vi "Lab Panel V5.25.vi"() -> ()   [LabVIEW 2017] (continued)
                            n3233 = Multiply(x=w5970, y=w5972) -> (x*y=w5971:dbl)
                          }
                        }
                        n3234 = local read "SIG LAB05-1"() -> (w5957:T2)
                        n3235 = Bundle By Name(cluster=w5957, "Tmp Live"=w5937, "Tmp Neut"=w5936) -> (w5956:T2)
                        n3236 = local read "SIG LAB05-2"() -> (w5955:T2)
                        n3237 = Bundle By Name(cluster=w5955, "Tmp Live"=w5933, "Tmp Neut"=w5932) -> (w5954:T2)
                        n3238 = local write "SIG LAB05-1"(w5956) -> ()
                        n3239 = local write "SIG LAB05-2"(w5954) -> ()
                      }
                    }
                  }
                }
              }
            }
          }
          frame #21 {
            # "write data to display panel"
            n3240 = global write "Global display 1.vi" "TEST 5-2"(w6009) -> ()
            n3241 = global write "Global display 1.vi" "TEST 4-2"(w6011) -> ()
            n3242 = global write "Global display 1.vi" "TEST 1-2"(w6017) -> ()
            n3243 = global write "Global display 1.vi" "TEST 3-1"(w6014) -> ()
            n3244 = global write "Global display 1.vi" "TEST 5-1"(w6010) -> ()
            n3245 = global write "Global display 1.vi" "TEST 1-1"(w6018) -> ()
            n3246 = global write "Global display 1.vi" "TEST 3-2"(w6013) -> ()
            n3247 = global write "Global display 1.vi" "TEST 4-1"(w6012) -> ()
            n3248 = global write "Global display 1.vi" "TEST 2-2"(w6015) -> ()
            n3249 = global write "Global display 1.vi" "TEST 2-1"(w6016) -> ()
            n3250 = global read "Global display 3.vi" "log 1-1"() -> (→"LOG LAB01-1":string)
            n3251 = global read "Global display 3.vi" "log 3-1"() -> (→"LOG LAB03-1":string)
            n3252 = global read "Global display 3.vi" "log 1-2"() -> (→"LOG LAB01-2":string)
            n3253 = property on="Tab Control 2" class="TabCtl (strict)"() -> ("Pages"=w6008:refnum<vi>[])  [unwired: 2 in, 2 out]
            n3254 = global read "Global display 3.vi" "log 2-1"() -> (→"LOG LAB02-1":string)
            n3255 = global read "Global display 3.vi" "log 2-2"() -> (→"LOG LAB02-2":string)
            n3256 = global read "Global display 3.vi" "log 4-2"() -> (→"LOG LAB04-2":string)
            n3257 = global read "Global display 3.vi" "log 5-2"() -> (→"LOG LAB05-2":string)
            n3258 = global read "Global display 3.vi" "log 5-1"() -> (→"LOG LAB05-1":string)
            n3259 = global read "Global display 3.vi" "log 4-1"() -> (→"LOG LAB04-1":string)
            n3260 = global read "Global display 3.vi" "log 3-2"() -> (→"LOG LAB03-2":string)
            n3261 = Index Array(array=w6008, index=8) -> (element=w6006:refnum<vi>)
            n3262 = property class="Page"(reference=w6006) -> ("PageVis"=w6005:bool)  [unwired: 1 in, 2 out]
            n3263 = global write "Global display 3.vi" "admin"(w6005) -> ()
            n3264 = local read "O/I  LAB05-2"() -> (w6059:bool)
            n3265 = local read "O/I  LAB05-1"() -> (w6060:bool)
            n3266 = local read "O/I  LAB03-2"() -> (w6063:bool)
            n3267 = local read "O/I  LAB04-2"() -> (w6061:bool)
            n3268 = local read "O/I  LAB04-1"() -> (w6062:bool)
            n3269 = local read "O/I  LAB03-1"() -> (w6064:bool)
            n3270 = local read "O/I  LAB01-2"() -> (w6067:bool)
            n3271 = local read "O/I  LAB01-1"() -> (w6068:bool)
            n3272 = local read "O/I  LAB02-1"() -> (w6066:bool)
            n3273 = local read "O/I  LAB02-2"() -> (w6065:bool)
            n3274 = global write "Global display 1.vi" "5-2 O/F"(w6059) -> ()
            n3275 = global write "Global display 1.vi" "5-1 O/F"(w6060) -> ()
            n3276 = global write "Global display 1.vi" "4-1 O/F"(w6062) -> ()
            n3277 = global write "Global display 1.vi" "4-2 O/F"(w6061) -> ()
            n3278 = global write "Global display 1.vi" "3-2 O/F"(w6063) -> ()
            n3279 = global write "Global display 1.vi" "3-1 O/F"(w6064) -> ()
            n3280 = global write "Global display 1.vi" "2-2 O/F"(w6065) -> ()
            n3281 = global write "Global display 1.vi" "2-1 O/F"(w6066) -> ()
            n3282 = global write "Global display 1.vi" "1-2 O/F"(w6067) -> ()
            n3283 = global write "Global display 1.vi" "1-1 O/F"(w6068) -> ()
            n3284 = local read "run lab05-2"() -> (w6049:bool)
            n3285 = local read "run lab04-1"() -> (w6052:bool)
            n3286 = local read "run lab04-2"() -> (w6051:bool)
            n3287 = local read "run lab05-1"() -> (w6050:bool)
            n3288 = local read "TEMP START LAB02-2"() -> (w5991:cluster{"TL":dbl, "TN":dbl})
            n3289 = local read "TEMP START LAB01-2"() -> (w5993:cluster{"TL":dbl, "TN":dbl})
            n3290 = local read "TEMP START LAB02-1"() -> (w5992:cluster{"TL":dbl, "TN":dbl})
            n3291 = local read "TEMP START LAB04-1"() -> (w5988:cluster{"TL":dbl, "TN":dbl})
            n3292 = local read "TEMP START LAB04-2"() -> (w5987:cluster{"TL":dbl, "TN":dbl})
            n3293 = local read "run lab03-2"() -> (w6053:bool)
            n3294 = local read "TEMP START LAB01-1"() -> (w5994:cluster{"TL":dbl, "TN":dbl})
            n3295 = local read "TEMP START LAB05-2"() -> (w5985:cluster{"TL":dbl, "TN":dbl})
            n3296 = local read "TEMP START LAB05-1"() -> (w5986:cluster{"TL":dbl, "TN":dbl})
            n3297 = local read "run lab02-1"() -> (w6056:bool)
            n3298 = local read "run lab03-1"() -> (w6054:bool)
            n3299 = local read "TEMP START LAB03-2"() -> (w5989:cluster{"TL":dbl, "TN":dbl})
            n3300 = local read "run lab01-2"() -> (w6057:bool)
            n3301 = local read "run lab02-2"() -> (w6055:bool)
            n3302 = local read "TEMP START LAB03-1"() -> (w5990:cluster{"TL":dbl, "TN":dbl})
            n3303 = local read "run lab01-1"() -> (w6058:bool)
            n3304 = global write "Global display 1.vi" "5-2 R/S"(w6049) -> ()
            n3305 = global write "Global display 1.vi" "5-1 R/S"(w6050) -> ()
            n3306 = global write "Global display 1.vi" "4-2 R/S"(w6051) -> ()
            n3307 = global write "Global display 1.vi" "4-1 R/S"(w6052) -> ()
            n3308 = global write "Global display 1.vi" "3-2 R/S"(w6053) -> ()
            n3309 = global write "Global display 1.vi" "1-2 R/S"(w6057) -> ()
            n3310 = global write "Global display 1.vi" "2-1 R/S"(w6056) -> ()
            n3311 = global write "Global display 1.vi" "3-1 R/S"(w6054) -> ()
            n3312 = global write "Global display 1.vi" "2-2 R/S"(w6055) -> ()
            n3313 = global write "Global display 1.vi" "1-1 R/S"(w6058) -> ()
            n3314 = global write "Global display 3.vi" "TEMP ST 05-2"(w5985) -> ()
            n3315 = global write "Global display 3.vi" "TEMP ST 05-1"(w5986) -> ()
            n3316 = global write "Global display 3.vi" "TEMP ST 03-2"(w5989) -> ()
            n3317 = global write "Global display 3.vi" "TEMP ST 04-2"(w5987) -> ()
            n3318 = global write "Global display 3.vi" "TEMP ST 01-1"(w5994) -> ()
            n3319 = global write "Global display 3.vi" "TEMP ST 01-2"(w5993) -> ()
            n3320 = global write "Global display 3.vi" "TEMP ST 04-1"(w5988) -> ()
            n3321 = global write "Global display 3.vi" "TEMP ST 02-1"(w5992) -> ()
            n3322 = global write "Global display 3.vi" "TEMP ST 02-2"(w5991) -> ()
            n3323 = global write "Global display 3.vi" "TEMP ST 03-1"(w5990) -> ()
            n3324 = local read "DISP LAB04-2"() -> (w6041:T4)
            n3325 = local read "DISP LAB05-1"() -> (w6040:T4)
            n3326 = local read "DISP LAB04-1"() -> (w6042:T4)
            n3327 = local read "DISP LAB05-2"() -> (w6039:T4)
            n3328 = local read "DISP LAB03-1"() -> (w6044:T4)
            n3329 = local read "DISP LAB03-2"() -> (w6043:T4)
            n3330 = local read "DISP LAB01-2"() -> (w6047:T4)
            n3331 = local read "DISP LAB02-1"() -> (w6046:T4)
            n3332 = local read "DISP LAB02-2"() -> (w6045:T4)
            n3333 = local read "DISP LAB01-1"() -> (w6048:T4)
            n3334 = local read "TEMP RISE LAB05-1"() -> (w5976:cluster{"TL":dbl, "TN":dbl})
            n3335 = local read "TEMP RISE LAB05-2"() -> (w5975:cluster{"TL":dbl, "TN":dbl})
            n3336 = local read "TEMP RISE LAB04-2"() -> (w5977:cluster{"TL":dbl, "TN":dbl})
            n3337 = local read "TEMP RISE LAB04-1"() -> (w5978:cluster{"TL":dbl, "TN":dbl})
            n3338 = local read "TEMP RISE LAB03-2"() -> (w5979:cluster{"TL":dbl, "TN":dbl})
            n3339 = local read "TEMP RISE LAB03-1"() -> (w5980:cluster{"TL":dbl, "TN":dbl})
            n3340 = local read "TEMP RISE LAB01-2"() -> (w5983:cluster{"TL":dbl, "TN":dbl})
            n3341 = local read "TEMP RISE LAB02-2"() -> (w5981:cluster{"TL":dbl, "TN":dbl})
            n3342 = local read "TEMP RISE LAB01-1"() -> (w5984:cluster{"TL":dbl, "TN":dbl})
            n3343 = local read "TEMP RISE LAB02-1"() -> (w5982:cluster{"TL":dbl, "TN":dbl})
            n3344 = global write "Global display 2.vi" "DISP LAB05-1"(w6040) -> ()
            n3345 = global write "Global display 2.vi" "DISP LAB05-2"(w6039) -> ()
            n3346 = global write "Global display 2.vi" "DISP LAB04-2"(w6041) -> ()
            n3347 = global write "Global display 2.vi" "DISP LAB02-1"(w6046) -> ()
            n3348 = global write "Global display 2.vi" "DISP LAB02-2"(w6045) -> ()
            n3349 = global write "Global display 2.vi" "DISP LAB04-1"(w6042) -> ()
            n3350 = global write "Global display 2.vi" "DISP LAB01-2"(w6047) -> ()
            n3351 = global write "Global display 2.vi" "DISP LAB01-1"(w6048) -> ()
            n3352 = global write "Global display 2.vi" "DISP LAB03-1"(w6044) -> ()
            n3353 = global write "Global display 2.vi" "DISP LAB03-2"(w6043) -> ()
            n3354 = global write "Global display 3.vi" "TEMP RS 05-2"(w5975) -> ()
            n3355 = global write "Global display 3.vi" "TEMP RS 05-1"(w5976) -> ()
            n3356 = global write "Global display 3.vi" "TEMP RS 03-2"(w5979) -> ()
            n3357 = global write "Global display 3.vi" "TEMP RS 02-1"(w5982) -> ()
            n3358 = global write "Global display 3.vi" "TEMP RS 02-2"(w5981) -> ()
            n3359 = global write "Global display 3.vi" "TEMP RS 04-2"(w5977) -> ()
            n3360 = global write "Global display 3.vi" "TEMP RS 01-2"(w5983) -> ()
            n3361 = global write "Global display 3.vi" "TEMP RS 03-1"(w5980) -> ()
            n3362 = global write "Global display 3.vi" "TEMP RS 04-1"(w5978) -> ()
            n3363 = global write "Global display 3.vi" "TEMP RS 01-1"(w5984) -> ()
            n3364 = local read "SET LAB05-2"() -> (w6029:T5)
            n3365 = local read "SET LAB05-1"() -> (w6030:T5)
            n3366 = local read "SET LAB04-1"() -> (w6032:T5)
            n3367 = local read "SET LAB04-2"() -> (w6031:T5)
            n3368 = local read "SET LAB03-1"() -> (w6034:T5)
            n3369 = local read "SET LAB03-2"() -> (w6033:T5)
            n3370 = local read "SET LAB02-2"() -> (w6035:T5)
            n3371 = local read "SET LAB01-2"() -> (w6037:T5)
            n3372 = local read "SET LAB02-1"() -> (w6036:T5)
            n3373 = local read "SET LAB01-1"() -> (w6038:T5)
            n3374 = global write "Global display 2.vi" "SET LAB05-2"(w6029) -> ()
            n3375 = global write "Global display 2.vi" "SET LAB05-1"(w6030) -> ()
            n3376 = global write "Global display 2.vi" "SET LAB04-1"(w6032) -> ()
            n3377 = global write "Global display 2.vi" "SET LAB04-2"(w6031) -> ()
            n3378 = global write "Global display 2.vi" "SET LAB03-2"(w6033) -> ()
            n3379 = global write "Global display 2.vi" "SET LAB02-2"(w6035) -> ()
            n3380 = global write "Global display 2.vi" "SET LAB03-1"(w6034) -> ()
            n3381 = global write "Global display 2.vi" "SET LAB01-2"(w6037) -> ()
            n3382 = global write "Global display 2.vi" "SET LAB01-1"(w6038) -> ()
            n3383 = global write "Global display 2.vi" "SET LAB02-1"(w6036) -> ()
            n3384 = local read "RESULT LAB01-1"() -> (w6028:bool)
            n3385 = local read "RESULT LAB03-2"() -> (w6023:bool)
            n3386 = local read "RESULT LAB04-1"() -> (w6022:bool)
            n3387 = local read "RESULT LAB04-2"() -> (w6021:bool)
            n3388 = local read "RESULT LAB02-2"() -> (w6025:bool)
            n3389 = local read "RESULT LAB01-2"() -> (w6027:bool)
            n3390 = local read "RESULT LAB02-1"() -> (w6026:bool)
            n3391 = local read "RESULT LAB03-1"() -> (w6024:bool)
            n3392 = local read "RESULT LAB05-1"() -> (w6020:bool)
            n3393 = local read "RESULT LAB05-2"() -> (w6019:bool)
            n3394 = global write "Global display 2.vi" "RESULT LAB05-1"(w6020) -> ()
            n3395 = global write "Global display 2.vi" "RESULT LAB01-2"(w6027) -> ()
            n3396 = global write "Global display 2.vi" "RESULT LAB03-2"(w6023) -> ()
            n3397 = global write "Global display 2.vi" "RESULT LAB04-1"(w6022) -> ()
            n3398 = global write "Global display 2.vi" "RESULT LAB04-2"(w6021) -> ()
            n3399 = global write "Global display 2.vi" "RESULT LAB05-2"(w6019) -> ()
            n3400 = global write "Global display 2.vi" "RESULT LAB03-1"(w6024) -> ()
            n3401 = global write "Global display 2.vi" "RESULT LAB02-1"(w6026) -> ()
            n3402 = global write "Global display 2.vi" "RESULT LAB02-2"(w6025) -> ()
            n3403 = global write "Global display 2.vi" "RESULT LAB01-1"(w6028) -> ()
          }
          frame #22 {
            # "simulate values"
            n3404 = global write "Global display 4.vi" "LAB deg C"("LAB deg C") -> ()
          }
          frame #23 {
            # "end main and display program"
            n3405 = stacked-sequence {
              seq-local: [_ w6074 _] -> [_ _ w6078]
              tunnel: w6071 -> [w6072 _ _]
              tunnel: w6070 -> [_ _ w6076]
              frame #0 {
                n3406 = case shown="True" w6072 {
                  frame False {
                  }
                  frame True {
                    n3407 = One Button Dialog(message="Excessive number of USB \nresets done, re-start program.") -> ()  [unwired: 1 in, 1 out]
                  }
                }
              }
              frame #1 {
                # "check for reset error"
                n3408 = local read "Reset Error"() -> (w6074:bool)
                n3409 = case shown="True" w6074 {
                  frame False {
                  }
                  frame True {
                    n3410 = One Button Dialog(message="USB ERROR, program will be stopped.\nClose program, close windows, switch panel off\nand re power panel. If error persists seek help.") -> ()  [unwired: 1 in, 1 out]
                  }
                }
              }
              frame #2 {
                # "end labview session"
                n3411 = case shown="True" w6076 {
                  frame False {
                  }
                  frame True {
                    n3412 = local read "AI Task2"() -> (w6082:dbl)
                    n3413 = local read "AI Task1"() -> (w6081:dbl)
                    n3414 = local read "AI Task0"() -> (w6080:dbl)
                    n3415 = call "sub vi - AI USB4704 (3)  Close Task v2.vi"(0:w6080, 5:w6081, 7:w6082) -> ()  [unwired: 13 in]
                  }
                }
                n3416 = Or(x=w6078, y="stop all") -> (x .or. y?=w6077:bool)
                n3417 = case shown="True" w6077 {
                  frame False {
                  }
                  frame True {
                    n3418 = stacked-sequence {
                      frame #0 {
                        n3419 = local read "AI Task2"() -> (w6083:dbl)
                        n3420 = local read "AI Task1"() -> (w6084:dbl)
                        n3421 = local read "AI Task0"() -> (w6085:dbl)
                        n3422 = call "sub vi - AI USB4704 (3)  Close Task v2.vi"(0:w6085, 5:w6084, 7:w6083) -> ()  [unwired: 13 in]
                      }
                      frame #1 {
                        w6086 = TRUE
                        n3423 = global write "Global display 1.vi" "stop disp"(w6086) -> ()
                        n3424 = Quit LabVIEW(quit? (T)=w6086) -> ()
                      }
                    }
                  }
                }
              }
            }
          }
        }
        n3425 = node-c288() -> ()  [unwired: 1 in, 1 out]
        "loops" <- w342
      }
      n3426 = node-c288(w315) -> ()  [unwired: 1 out]
    }
  }
